vi "Set Color.vi"(8 "Error In":errorcluster, 10 "Color":u32(colorbox), 11 "Display Element in":refnum<class "Display Element.lvclass">) -> (0 "Error Out":errorcluster, 3 "Display Element out":refnum<class "Display Element.lvclass">)   [LabVIEW 2019, in "Display Element.lvclass"]
uses:
  Display Element.lvclass
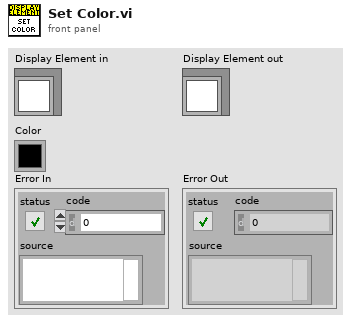
[diagram p1: front panel]
types:
  T1 = typedef "Display Element.lvclass/Data.ctl" = cluster{"Color":u32, "Layer":u32, "Tag":string, "Position":T2, "Force":T2, "Delete If Outside Bounds":bool}
  T2 = typedef "Display Element.lvclass/Vector.ctl" = cluster{"X":i32, "Y":i32}
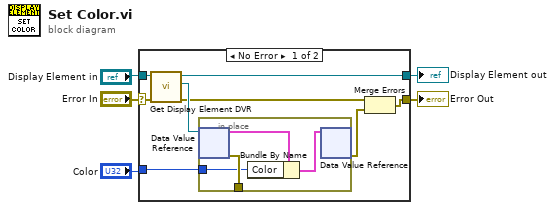
[diagram p0: block diagram]
diagram:
  n1 = case shown="No Error" "Error In" {
    selector: "Error In" -> [w9 w18]
    tunnel: [w12 w18] -> w2
    tunnel: [w7 w19] -> w1
    tunnel: "Display Element in" -> [w10 w19]
    tunnel: "Color" -> [w11 _]
    frame No Error {
      n2 = call "Get Display Element DVR.vi"("Error In"=w9, "Display Element In"=w10) -> ("Error Out"=w6:errorcluster, "DVR"=w8:refnum<data-value>, "Display Element Out"=w7:refnum<class "Display Element.lvclass">)  [unwired: 7 in]
      n3 = in-place {
        in-place-border: [w17] -> _
        in-place-border: w11 -> [w14]
        n4 = in-place-dvr #1(w8) -> (w16:T1, w17:errorcluster)
        n5 = Bundle By Name(cluster=w16, "Color"=w14) -> (w15:T1)
        n6 = in-place-dvr #1(w15) -> (w13:errorcluster)  [unwired: 1 out]
      }
      n7 = Merge Errors(w6, w13) -> (w12:errorcluster)
    }
    frame Error {
    }
  }
  "Display Element out" <- w1
  "Error Out" <- w2
